vi "observacao_0MQ.vi"() -> ()   [LabVIEW 2012, in "Shared_160.lvlib"] (continued)
                    n1919 = property on="Sent_EspLampCass" class="Bool (strict)"("Disabled"=w2415) -> ()  [unwired: 2 in, 2 out]
                    n1920 = property on="Ne" class="Bool (strict)"("Disabled"=w2415) -> ()  [unwired: 2 in, 2 out]
                    n1921 = property on="He-Ar" class="Bool (strict)"("Disabled"=w2415) -> ()  [unwired: 2 in, 2 out]
                    n1922 = Add(x=w2416, y=u8 4) -> (x+y=w2418:u8)
                    n1923 = Greater Or Equal?(x=w2418, y=u8 100 ("x")) -> (x >= y?=w2419:bool)
                    n1924 = case shown="True" w2419 {
                      selector: w2419 -> [_ w2423]
                      tunnel: w2418 -> [w2422 _]
                      frame False {
                        n1925 = local write "SlideEcass"(w2422) -> ()
                        n1926 = property on="SlideEcass" class="Slide (strict)"("Fill Color"=u32 16750950 ("color(black)")) -> ()  [unwired: 2 in, 2 out]
                      }
                      frame True {
                        n1927 = local write "SlideEcass"(u8 92 ("Slide")) -> ()
                        n1928 = property on="stopEcass" class="Bool"("Visible"=w2423) -> ()  [unwired: 2 in, 2 out]
                        n1929 = property on="SlideEcass" class="Slide (strict)"("Fill Color"=u32 16724787 ("color(black)")) -> ()  [unwired: 2 in, 2 out]
                      }
                    }
                  }
                }
              }
              frame "Eucalyp." {
                # "Eucalyptus"
              }
              frame "Cam 1" {
                w2467 = 10
                w2474 = u16 15 items=["Alarme", "Atencao", "Erro", "Ocupado", "PosSecund", "PosConj#3", "MovFoco", "MovCjto#3", "Mov#4", "Mov#3", "Mov#2", "EspLamp", "HE", "NE", "EspLampRepouso", "EspLampCalibra"] ("NomeStatus")
                w2475 = u16 14 items=["Alarme", "Atencao", "Erro", "Ocupado", "PosSecund", "PosConj#3", "MovFoco", "MovCjto#3", "Mov#4", "Mov#3", "Mov#2", "EspLamp", "HE", "NE", "EspLampRepouso", "EspLampCalibra"] ("NomeStatus")
                w2476 = u16 11 items=["Alarme", "Atencao", "Erro", "Ocupado", "PosSecund", "PosConj#3", "MovFoco", "MovCjto#3", "Mov#4", "Mov#3", "Mov#2", "EspLamp", "HE", "NE", "EspLampRepouso", "EspLampCalibra"] ("NomeStatus")
                # "MUDANÇA:\nDESABILITA COMANDOS\nDE MOV. DO ESPELHO.\nRemover na implantação\ndefinitiva da CAM1."
                # "CAM 1"
                n1930 = event shown="[1] \"Mover/Parar\": Value Change" {
                  selector: _ -> [_ _ _ _]
                  dyn-events: _ -> [_ _ _ _]
                  timeout: w2467 -> [_ _ _ _]
                  tunnel: ["timeout" ("Comando") w2493 w2499 w2505] -> w2460
                  event Timeout {
                    n1931 = event-data() -> ()  [unwired: 1 in, 2 out]
                  }
                  event "Mover/Parar": Value Change {
                    w2495 = u16 3 items=["ZERO", "AH", "DEC", "TUBO", "CUP"] ("Controlador")
                    n1932 = event-data() -> ("NewVal"=w2496:bool)  [unwired: 1 in, 4 out]
                    n1933 = case shown="True" w2496 {
                      tunnel: ["PARAR" ("Comando") "GIRAR" ("Comando")] -> w2493
                      frame False {
                      }
                      frame True {
                      }
                    }
                    n1934 = call "Monta Comando.vi"("Comando"=w2493, "Dispositivo"="ESP_CAMP", "Controlador"=w2495) -> ()  [unwired: 4 in, 3 out]
                  }
                  event "Sentido": Value Change {
                    w2500 = u16 3 items=["ZERO", "AH", "DEC", "TUBO", "CUP"] ("Controlador")
                    n1935 = event-data() -> ("NewVal"=w2502:bool)  [unwired: 1 in, 4 out]
                    n1936 = case shown="False" w2502 {
                      tunnel: ["RECUAR" "AVANCAR"] -> w2499
                      frame False {
                      }
                      frame True {
                      }
                    }
                    n1937 = call "Monta Comando.vi"("Comando"=w2499, "Dispositivo"="ESP_CAMP", "Controlador"=w2500) -> ()  [unwired: 4 in, 3 out]
                  }
                  event "Velocidade": Value Change {
                    w2507 = u16 3 items=["ZERO", "AH", "DEC", "TUBO", "CUP"] ("Controlador")
                    n1938 = event-data() -> ("NewVal"=w2508:bool)  [unwired: 1 in, 4 out]
                    n1939 = case shown="True" w2508 {
                      tunnel: ["AUMENTAR" "DIMINUIR"] -> w2505
                      frame False {
                      }
                      frame True {
                      }
                    }
                    n1940 = call "Monta Comando.vi"("Comando"=w2505, "Dispositivo"="ESP_CAMP", "Controlador"=w2507) -> ()  [unwired: 4 in, 3 out]
                  }
                }
                "Comando" <- w2460
                n1941 = event shown="[1] \"Sent_EspDesvFeixe\": Value Change" {
                  selector: _ -> [_ _ _]
                  dyn-events: _ -> [_ _ _]
                  timeout: w2467 -> [_ _ _]
                  event Timeout {
                    n1942 = event-data() -> ()  [unwired: 1 in, 2 out]
                  }
                  event "Sent_EspDesvFeixe": Value Change {
                    n1943 = event-data() -> ()  [unwired: 1 in, 4 out]
                    n1944 = case shown="1" "Disabled" {
                      tunnel: ["RECUAR" ("Comando") "AVANCAR" ("Comando")] -> w2514
                      tunnel: ["ESP_LAMP" ("Dispositivo") "ESP_LAMP" ("Dispositivo")] -> w2513
                      frame 0, Default {
                        # "Case False (Default) em\noperação normal, com o\nbotão Sent_EspDesvFeixe\nligado ao ? deste case."
                      }
                      frame 1 {
                        # "CaseTrue. Cf. nota no case 0"
                        n1945 = property on="SlideCam1" class="Slide (strict)"("Visible"=TRUE) -> ()  [unwired: 2 in, 2 out]
                        n1946 = property on="stopCam1" class="Bool"("Visible"=FALSE) -> ()  [unwired: 2 in, 2 out]
                        "SlideCam1" <- u8 5 ("Slide 2")
                      }
                    }
                    n1947 = case shown="True" "Case Constant\n(See Context Help) 9" {
                      tunnel: w2514 -> [_ w2517]
                      tunnel: w2513 -> [_ w2516]
                      frame False {
                      }
                      frame True {
                        w2515 = u16 3 items=["ZERO", "AH", "DEC", "TUBO", "CUP"] ("Controlador")
                        n1948 = call "Monta Comando.vi"("Comando"=w2517, "Dispositivo"=w2516, "Controlador"=w2515) -> ()  [unwired: 4 in, 3 out]
                      }
                    }
                  }
                  event "Go_filtro": Value Change {
                    n1949 = event-data() -> ()  [unwired: 1 in, 6 out]
                    n1950 = case shown="True" "Go_filtro" {
                      frame False {
                      }
                      frame True {
                        (unwired) "ZERO: Porta serial da CAM1"
                        w2526 = u16 0 items=["ZERO", "AH", "DEC", "TUBO", "CUP"] ("Controlador")
                        n1951 = call "Monta Comando.vi"("Set Point"="Filtro", "Controlador"=w2526) -> ()  [unwired: 5 in, 3 out]
                      }
                    }
                  }
                }
                n1952 = case shown="False" "Sentido" {
                  tunnel: [TRUE FALSE] -> w2465
                  tunnel: [FALSE TRUE] -> w2464
                  frame False {
                  }
                  frame True {
                  }
                }
                "Recuar" <- w2465
                "Avancar" <- w2464
                n1953 = case shown="False" "Velocidade" {
                  tunnel: [TRUE FALSE] -> w2462
                  tunnel: [FALSE TRUE] -> w2461
                  frame False {
                  }
                  frame True {
                  }
                }
                "Rapido" <- w2462
                "Lento" <- w2461
                n1954 = call "Bit Status TUBO.vi"("NomeStatus"=w2476) -> ("StatBit"=w2473:bool)
                n1955 = call "Bit Status TUBO.vi"("NomeStatus"=w2475) -> ("StatBit"=w2472:bool)
                n1956 = call "Bit Status TUBO.vi"("NomeStatus"=w2474) -> ("StatBit"=w2471:bool)
                n1957 = Not(x=w2473) -> (.not. x?=w2482:bool)
                n1958 = And(x=w2473, y=w2472) -> (x .and. y?=w2478:bool)
                "LedRepCam1" <- w2478
                n1959 = Or(x=w2472, y=w2471) -> (x .or. y?=w2483:bool)
                n1960 = And(x=w2473, y=w2471) -> (x .and. y?=w2477:bool)
                "LedCalCam1" <- w2477
                n1961 = property on="SlideCam1" class="Slide (strict)"() -> ("Visible"=w2480:bool)  [unwired: 2 in, 2 out]
                n1962 = Or(x=w2478, y=w2477) -> (x .or. y?=w2481:bool)
                n1963 = And(x=w2482, y=w2483) -> (x .and. y?=w2469:bool)
                n1964 = And(x="Case Constant\n(See Context Help) 10", y=w2469) -> (x .and. y?=w2470:bool)
                n1965 = case shown="True" "Case Constant\n(See Context Help) 10" {
                  frame False {
                  }
                  frame True {
                    w2541 = FALSE
                    w2544 = u16 3 items=["ZERO", "AH", "DEC", "TUBO", "CUP"] ("Controlador")
                    w2542 = u8 0 ("Disabled")
                    n1966 = call "Monta Comando.vi"("Comando"="DESLIGAR", "Dispositivo"="ESP_LAMP", "Controlador"=w2544) -> ()  [unwired: 4 in, 3 out]
                    n1967 = property on="Sent_EspDesvFeixe" class="Bool (strict)"("Disabled"=w2542) -> ()  [unwired: 2 in, 2 out]
                    n1968 = property on="Go_filtro" class="Bool"("Disabled"=w2542) -> ()  [unwired: 2 in, 2 out]
                    n1969 = property on="stopCam1" class="Bool"("Visible"=w2541) -> ()  [unwired: 2 in, 2 out]
                    n1970 = property on="SlideCam1" class="Slide (strict)"("Visible"=w2541) -> ()  [unwired: 2 in, 2 out]
                  }
                }
                n1971 = case shown="True" w2470 {
                  frame False {
                  }
                  frame True {
                    w2529 = u8 2 ("Disabled")
                    n1972 = local read "SlideCam1"() -> (w2528:u8)
                    n1973 = Add(x=w2528, y=u8 5) -> (x+y=w2530:u8)
                    n1974 = property on="Sent_EspDesvFeixe" class="Bool (strict)"("Disabled"=w2529) -> ()  [unwired: 2 in, 2 out]
                    n1975 = property on="Go_filtro" class="Bool"("Disabled"=w2529) -> ()  [unwired: 2 in, 2 out]
                    n1976 = Greater Or Equal?(x=w2530, y=u8 100 ("x")) -> (x >= y?=w2532:bool)
                    n1977 = case shown="True" w2532 {
                      selector: w2532 -> [_ w2536]
                      tunnel: w2530 -> [w2534 _]
                      frame False {
                        n1978 = local write "SlideCam1"(w2534) -> ()
                        n1979 = property on="SlideCam1" class="Slide (strict)"("Fill Color"=u32 16750950 ("color(black)")) -> ()  [unwired: 2 in, 2 out]
                      }
                      frame True {
                        n1980 = property on="stopCam1" class="Bool"("Visible"=w2536) -> ()  [unwired: 2 in, 2 out]
                        n1981 = local write "SlideCam1"(u8 90 ("Slide 2")) -> ()
                        n1982 = property on="SlideCam1" class="Slide (strict)"("Fill Color"=u32 16724787 ("color(black)")) -> ()  [unwired: 2 in, 2 out]
                      }
                    }
                  }
                }
                n1983 = And(x=w2480, y=w2481) -> (x .and. y?=w2479:bool)
                n1984 = case shown="True" w2479 {
                  frame False {
                  }
                  frame True {
                    w2540 = u8 0 ("Disabled")
                    n1985 = property on="Go_filtro" class="Bool"("Disabled"=w2540) -> ()  [unwired: 2 in, 2 out]
                    n1986 = property on="Sent_EspDesvFeixe" class="Bool (strict)"("Disabled"=w2540) -> ()  [unwired: 2 in, 2 out]
                    n1987 = property on="SlideCam1" class="Slide (strict)"("Visible"=FALSE) -> ()  [unwired: 2 in, 2 out]
                  }
                }
              }
              frame "Cam 2" {
                # "Cam 2"
              }
              frame "Cam IV." {
                # "Cam IV"
              }
              frame "Polarim." {
                # "Polarimetro"
              }
              frame "Fotrap" {
                # "Fotrap"
              }
              frame "Coude", Default {
                # "COUDE"
                n1988 = stacked-sequence {
                  frame #0 {
                    w2548 = u16 5 items=["Alarme", "Atencao", "Erro", "Ocupado", "Stop#3", "Cass#3", "MovFoco", "PosSecund", "Mov#2", "Mov#3", "Mov#4", "EspLamp", "HE", "NE", "EspLampRepouso", "EspLampCalibra"] ("NomeStatus")
                    w2547 = u16 7 items=["Alarme", "Atencao", "Erro", "Ocupado", "Stop#3", "Cass#3", "MovFoco", "PosSecund", "Mov#2", "Mov#3", "Mov#4", "EspLamp", "HE", "NE", "EspLampRepouso", "EspLampCalibra"] ("NomeStatus")
                    n1989 = local read "EspAtual"() -> (w2550:string)
                    n1990 = case shown="\"A\"" w2550 {
                      frame "X", Default {
                        w2551 = FALSE
                        n1991 = local write "ledVisivel"(w2551) -> ()
                        n1992 = local write "ledAzul"(w2551) -> ()
                        n1993 = local write "ledVermelho"(w2551) -> ()
                      }
                      frame "M" {
                        w2552 = FALSE
                        n1994 = local write "ledAzul"(w2552) -> ()
                        n1995 = local write "ledVermelho"(w2552) -> ()
                        n1996 = local write "ledVisivel"(w2552) -> ()
                      }
                      frame "A" {
                        # "Espelho A --> Azul\nEspelho B --> Visível\nEspelho C --> Vermelho"
                        n1997 = local write "ledVermelho"(FALSE) -> ()
                        n1998 = local write "ledVisivel"(FALSE) -> ()
                        n1999 = local write "ledAzul"(TRUE) -> ()
                      }
                      frame "B" {
                        # "Espelho A --> Azul\nEspelho B --> Visível\nEspelho C --> Vermelho"
                        n2000 = local write "ledVermelho"(FALSE) -> ()
                        n2001 = local write "ledVisivel"(TRUE) -> ()
                        n2002 = local write "ledAzul"(FALSE) -> ()
                      }
                      frame "C" {
                        # "Espelho A --> Azul\nEspelho B --> Visível\nEspelho C --> Vermelho"
                        n2003 = local write "ledVermelho"(TRUE) -> ()
                        n2004 = local write "ledVisivel"(FALSE) -> ()
                        n2005 = local write "ledAzul"(FALSE) -> ()
                      }
                    }
                    n2006 = call "Bit Status TUBO.vi"("NomeStatus"=w2548) -> ("StatBit"=→"Cjto_3":bool)
                    n2007 = call "Bit Status TUBO.vi"("NomeStatus"=w2547) -> ("StatBit"=→"PosSecundario":bool)
                  }
                  frame #1 {
                    w2572 = u16 5 items=["Alarme", "Atencao", "Erro", "Ocupado", "Stop#3", "Cass#3", "MovFoco", "PosSecund", "Mov#2", "Mov#3", "Mov#4", "EspLamp", "HE", "NE", "EspLampRepouso", "EspLampCalibra"] ("NomeStatus")
                    w2577 = u16 8 items=["Alarme", "Atencao", "Erro", "Ocupado", "Stop#3", "Cass#3", "MovFoco", "PosSecund", "Mov#2", "Mov#3", "Mov#4", "EspLamp", "HE", "NE", "EspLampRepouso", "EspLampCalibra"] ("NomeStatus")
                    w2578 = u16 9 items=["Alarme", "Atencao", "Erro", "Ocupado", "Stop#3", "Cass#3", "MovFoco", "PosSecund", "Mov#2", "Mov#3", "Mov#4", "EspLamp", "HE", "NE", "EspLampRepouso", "EspLampCalibra"] ("NomeStatus")
                    w2579 = u16 10 items=["Alarme", "Atencao", "Erro", "Ocupado", "Stop#3", "Cass#3", "MovFoco", "PosSecund", "Mov#2", "Mov#3", "Mov#4", "EspLamp", "HE", "NE", "EspLampRepouso", "EspLampCalibra"] ("NomeStatus")
                    w2590 = u16 4 items=["Alarme", "Atencao", "Erro", "Ocupado", "Stop#3", "Cass#3", "MovFoco", "PosSecund", "Mov#2", "Mov#3", "Mov#4", "EspLamp", "HE", "NE", "EspLampRepouso", "EspLampCalibra"] ("NomeStatus")
                    w2591 = u16 3 items=["Alarme", "Atencao", "Erro", "Ocupado", "Stop#3", "Cass#3", "MovFoco", "PosSecund", "Mov#2", "Mov#3", "Mov#4", "EspLamp", "HE", "NE", "EspLampRepouso", "EspLampCalibra"] ("NomeStatus")
                    # "CJTO#3 EM \nMOVIMENTO"
                    n2008 = local read "PosSecundario"() -> (w2570:bool)
                    n2009 = call "Bit Status TUBO.vi"("NomeStatus"=w2572) -> ("StatBit"=w2569:bool)
                    n2010 = call "Bit Status TUBO.vi"("NomeStatus"=w2590) -> ("StatBit"=w2568:bool)
                    n2011 = call "Bit Status TUBO.vi"("NomeStatus"=w2591) -> ("StatBit"=w2566:bool)
                    n2012 = call "Bit Status TUBO.vi"("NomeStatus"=w2577) -> ("StatBit"=w2583:bool)
                    "#2" <- w2583
                    n2013 = call "Bit Status TUBO.vi"("NomeStatus"=w2578) -> ("StatBit"=w2582:bool)
                    "#3" <- w2582
                    n2014 = call "Bit Status TUBO.vi"("NomeStatus"=w2579) -> ("StatBit"=w2581:bool)
                    "#4" <- w2581
                    n2015 = Not Equal?(x=w2570, y=w2569) -> (x != y?=w2571:bool)
                    n2016 = Not(x=w2568) -> (.not. x?=w2564:bool)
                    n2017 = And(x=w2571, y=w2568) -> (x .and. y?=w2565:bool)
                    n2018 = Compound Arithmetic op=OR(w2583, w2582, w2581) -> (w2580:bool)
                    n2019 = Compound Arithmetic op=OR(w2565, w2564, w2566) -> (w2567:bool)
                    n2020 = property on="Cjto_3" class="Bool (strict)"("Blinking"=w2565) -> ()  [unwired: 2 in, 2 out]
                    n2021 = property on="PosSecundario" class="Bool (strict)"("Blinking"=w2565) -> ()  [unwired: 2 in, 2 out]
                    n2022 = case shown="True" w2567 {
                      tunnel: [T6."Page Enabled" ("Page Enabled State") T6."Page Disabled" ("Page Enabled State")] -> w2562
                      tunnel: [u8 0 ("Disabled") u8 2 ("Disabled")] -> w2576
                      frame False {
                      }
                      frame True {
                      }
                    }
                    n2023 = property on="MENSAGEM" class="Str"("Visible"=w2564, "Blinking"=w2564) -> ()  [unwired: 2 in, 2 out]
                    n2024 = case shown="True" w2580 {
                      tunnel: w2576 -> [w2595 _]
                      tunnel: [w2595 u8 2 ("Disabled")] -> w2575
                      tunnel: [FALSE TRUE] -> w2574
                      tunnel: [FALSE ("Blinking") TRUE ("Blinking")] -> w2573
                      frame False {
                        n2025 = local write "MENSAGEM 2"("EM MOVIMENTO" ("MENSAGEM 2")) -> ()
                      }
                      frame True {
                        n2026 = local read "EndTime"() -> (w2604:u32)
                        n2027 = Tick Count (ms)() -> (millisecond timer value=w2603:u32)
                        n2028 = Subtract(x=w2604, y=w2603) -> (x-y=w2602:u32)
                        n2029 = Divide(x=w2602, y=u32 1000) -> (x/y=w2599:dbl)
                        n2030 = To Unsigned Long Integer(number=w2599) -> (unsigned 32bit integer=w2600:u32)
                        n2031 = Number To Decimal String(number=w2600) -> (decimal integer string=w2597:string)  [unwired: 1 in]
                        n2032 = Concatenate Strings("EM MOVIMENTO " ("MENSAGEM 2"), w2597) -> (w2598:string)
                        n2033 = local write "MENSAGEM 2"(w2598) -> ()
                      }
                    }
                    n2034 = property on="Setup, Pointing & Guiding" class="TabCtl (strict)"() -> ("Pages"=w2563:refnum<vi>[])  [unwired: 2 in, 2 out]
                    n2035 = Index Array(array=w2563, index=4) -> (element=w2586:refnum<vi>)
                    n2036 = Index Array(array=w2563, index=5) -> (element=w2589:refnum<vi>)
                    n2037 = property class="Page"(reference=w2586, "Page Enabled State"=w2562) -> ()  [unwired: 1 in, 2 out]
                    n2038 = property class="Page"(reference=w2589, "Page Enabled State"=w2562) -> ()  [unwired: 1 in, 2 out]
                    n2039 = case shown="False" w2570 {
                      tunnel: [u8 0 ("Disabled") w2610] -> w2585
                      tunnel: w2575 -> [w2608 _]
                      tunnel: [w2608 w2610] -> w2584
                      frame False {
                        # "COUDE"
                      }
                      frame True {
                        w2610 = u8 2 ("Disabled")
                        # "CASS"
                      }
                    }
                    n2040 = property on="MENSAGEM 2" class="Str"("Visible"=w2574, "Blinking"=w2573) -> ()  [unwired: 2 in, 2 out]
                    n2041 = property on="ledAzul" class="Bool (strict)"("Disabled"=w2585) -> ()  [unwired: 2 in, 2 out]
                    n2042 = property on="ledVisivel" class="Bool (strict)"("Disabled"=w2585) -> ()  [unwired: 2 in, 2 out]
                    n2043 = property on="ledVermelho" class="Bool (strict)"("Disabled"=w2585) -> ()  [unwired: 2 in, 2 out]
                    n2044 = property on="Radio Buttons" class="RadioBtnsControl (strict)"("Disabled"=w2585) -> ()  [unwired: 2 in, 2 out]
                    n2045 = property on="#2" class="Bool (strict)"("Disabled"=w2585) -> ()  [unwired: 2 in, 2 out]
                    n2046 = property on="#3" class="Bool (strict)"("Disabled"=w2585) -> ()  [unwired: 2 in, 2 out]
                    n2047 = property on="#4" class="Bool (strict)"("Disabled"=w2585) -> ()  [unwired: 2 in, 2 out]
                    n2048 = property on="Go_Coudé" class="Bool"("Disabled"=w2584) -> ()  [unwired: 2 in, 2 out]
                  }
                  frame #2 {
                    n2049 = case shown="True" "Go_Coudé" {
                      frame False {
                        w2616 = u16 2 items=["Alarme", "Atencao", "Erro", "Ocupado", "Stop#3", "Cass#3", "MovFoco", "PosSecund", "Mov#2", "Mov#3", "Mov#4", "EspLamp", "HE", "NE", "EspLampRepouso", "EspLampCalibra"] ("NomeStatus")
                        w2617 = u16 3 items=["Alarme", "Atencao", "Erro", "Ocupado", "Stop#3", "Cass#3", "MovFoco", "PosSecund", "Mov#2", "Mov#3", "Mov#4", "EspLamp", "HE", "NE", "EspLampRepouso", "EspLampCalibra"] ("NomeStatus")
                        # "TRATA ERROS DO CONTROLADOR"
                        n2050 = call "Bit Status TUBO.vi"("NomeStatus"=w2616) -> ("StatBit"=w2619:bool)
                        n2051 = call "Bit Status TUBO.vi"("NomeStatus"=w2617) -> ("StatBit"=w2621:bool)
                        n2052 = Not(x=w2621) -> (.not. x?=w2620:bool)
                        n2053 = And(x=w2619, y=w2620) -> (x .and. y?=w2618:bool)
                        n2054 = case shown="True" w2618 {
                          frame False {
                          }
                          frame True {
                            w2624 = u16 3 items=["ZERO", "AH", "DEC", "TUBO", "CUP"] ("Controlador")
                            n2055 = call "Monta Comando.vi"("Comando"="ERROS", "Dispositivo"="PROG" ("Comando"), "Controlador"=w2624) -> ()  [unwired: 4 in, 3 out]
                          }
                        }
                      }
                      frame True {
                        w2625 = u16 3 items=["ZERO", "AH", "DEC", "TUBO", "CUP"] ("Controlador")
                        # "Enviar comando de \nmudar Espelho ABC"
                        n2056 = local read "EspAtual"() -> (w2631:string)
                        n2057 = case shown="\"Visível\"" "Radio Buttons" {
                          tunnel: ["C" ("Comando") "A" ("Comando") "B" ("Comando")] -> w2626
                          tunnel: w2631 -> [w2634 w2640 w2645]
                          tunnel: [w2633 w2639 w2646] -> w2628
                          frame "Vermelho" {
                            n2058 = case shown="\"A\"" w2634 {
                              tunnel: [u32 0 u32 60000 u32 35000] -> w2633
                              frame "C", Default {
                              }
                              frame "B" {
                              }
                              frame "A" {
                              }
                            }
                          }
                          frame "Azul", Default {
                            n2059 = case shown="\"C\"" w2640 {
                              tunnel: [u32 0 u32 35000 u32 60000] -> w2639
                              frame "A", Default {
                              }
                              frame "B" {
                              }
                              frame "C" {
                              }
                            }
                          }
                          frame "Visível" {
                            n2060 = case shown="\"C\"" w2645 {
                              tunnel: [u32 0 u32 60000 u32 35000] -> w2646
                              frame "B", Default {
                              }
                              frame "A" {
                              }
                              frame "C" {
                              }
                            }
                          }
                        }
                        n2061 = Tick Count (ms)() -> (millisecond timer value=w2630:u32)
                        n2062 = Add(x=w2630, y=w2628) -> (x+y=→"EndTime":u32)
                        n2063 = call "Monta Comando.vi"("Comando"=w2626, "Dispositivo"="ESPELHO" ("Comando"), "Controlador"=w2625) -> ()  [unwired: 4 in, 3 out]
                      }
                    }
                  }
                  frame #3 {
                    w2657 = 360.0
                    w2662 = 6.283185307179586
                    n2064 = global read "Global_Telescopio.vi" "guide_ang"() -> (w2672:string)
                    n2065 = global read "Global_Telescopio.vi" "guide_nor"() -> (w2673:string)
                    n2066 = global read "Global_Telescopio.vi" "AH_now"() -> (w2669:dbl)
                    n2067 = global read "Global_Telescopio.vi" "delta_now"() -> (w2670:dbl)
                    n2068 = Add(x=w2669, y=w2670) -> (x+y=w2661:dbl)
                    n2069 = Fract/Exp String To Number(string=w2672) -> (number=w2668:dbl)  [unwired: 3 in, 1 out]
                    n2070 = Fract/Exp String To Number(string=w2673) -> (number=w2671:dbl)  [unwired: 3 in, 1 out]
                    n2071 = Quotient & Remainder(x=w2661, y=w2662) -> (x-y*floor(x/y)=w2664:dbl)  [unwired: 1 out]
                    n2072 = Add(x=w2668, y=w2671) -> (x+y=w2653:dbl)
                    n2073 = Less Than 0?(x=w2664) -> (x < 0?=w2666:bool)
                    n2074 = case shown="True" w2666 {
                      tunnel: w2664 -> [w2674 w2677]
                      tunnel: [w2674 w2675] -> w2663
                      tunnel: w2662 -> [_ w2676]
                      frame False {
                      }
                      frame True {
                        n2075 = Add(x=w2677, y=w2676) -> (x+y=w2675:dbl)
                      }
                    }
                    n2076 = Add(x=124.0, y=w2653) -> (x+y=w2652:dbl)
                    n2077 = Multiply(x=w2663, y=57.29577951 ("x*y")) -> (x*y=w2660:dbl)
                    n2078 = Subtract(x=98.2, y=w2660) -> (x-y=w2659:dbl)
                    n2079 = Add(x=w2652, y=w2659) -> (x+y=w2656:dbl)
                    n2080 = Quotient & Remainder(x=w2656, y=w2657) -> (floor(x/y)=w2658:dbl)  [unwired: 1 out]
                    n2081 = Multiply(x=w2658, y=w2657) -> (x*y=w2655:dbl)
                    n2082 = Subtract(x=w2656, y=w2655) -> (x-y=→"Ang. Fenda":dbl)
                  }
                  frame #4 {
                    # "90"
                    # "270"
                    # "180"
                    # "0"
                    n2083 = event shown="[10] \"IronArc\": Value Change" {
                      selector: _ -> [_ _ _ _ _ _ _ _ _ _ _]
                      dyn-events: _ -> [_ _ _ _ _ _ _ _ _ _ _]
                      timeout: 10 -> [_ _ _ _ _ _ _ _ _ _ _]
                      event Timeout {
                        n2084 = event-data() -> ()  [unwired: 1 in, 2 out]
                        n2085 = stacked-sequence {
                          frame #0 {
                            n2086 = local read "parou 3"() -> (w2679:bool)
                            n2087 = case shown="True" w2679 {
                              frame False {
                              }
                              frame True {
                                n2088 = call "InstrumentControl.vi"("Input Message"="COUDE REDE POSICAO") -> ("Output Message"=w2682:string)  [unwired: 9 in, 1 out]
                                "Output Message" <- w2682
                                n2089 = Decimal String To Number(string=w2682) -> (number=w2681:i32)  [unwired: 2 in, 1 out]
                                n2090 = while {
                                shift-right: [w2685] -> w2680
                                shift-left: _ -> [w2689]
                                tunnel: w2681 -> [w2685]
                                stop <- TRUE stop-if-true
                                n2091 = Subtract(x=w2689, y=w2685) -> (x-y=w2688:i32)
                                n2092 = Absolute Value(x=w2688) -> (abs(x)=w2687:i32)
                                n2093 = Greater Or Equal?(x=w2687, y=1) -> (x >= y?=→"parou 3":bool)
                                }
                                "Posição Rede" <- w2680
                              }
                            }
                          }
                          frame #1 {
                            n2094 = local read "parou"() -> (w2692:bool)
                            n2095 = local read "parou 2"() -> (w2691:bool)
                            n2096 = case shown="True" w2691 {
                              frame False {
                              }
                              frame True {
                                # "Cada volta -> 10mm\nCada volta -> 4000counts\n1 count = 0,0025mm"
                                n2097 = call "InstrumentControl.vi"("Input Message"="COUDE ESPELHO POSICAO") -> ("Output Message"=w2699:string)  [unwired: 9 in, 1 out]
                                n2098 = Fract/Exp String To Number(string=w2699) -> (number=w2698:dbl)  [unwired: 3 in, 1 out]
                                n2099 = while {
                                shift-right: [w2711] -> w2694
                                shift-left: _ -> [w2712]
                                tunnel: w2698 -> [w2711]
                                tunnel: [w2707] -> w2693
                                stop <- TRUE stop-if-true
                                n2100 = Subtract(x=w2712, y=w2711) -> (x-y=w2710:dbl)
                                n2101 = Absolute Value(x=w2710) -> (abs(x)=w2709:dbl)
                                n2102 = Greater Or Equal?(x=w2709, y=0.02) -> (x >= y?=w2707:bool)
                                "parou 2" <- w2707
                                }
                                "Posição Espelho" <- w2694
                                n2103 = case shown="False" w2693 {
                                frame False {
                                n2104 = call "InstrumentControl.vi"("Input Message"="COUDE SERIAL CHAVEAR OFF") -> ()  [unwired: 9 in, 2 out]
                                }
                                frame True {
                                }
                                }
                                n2105 = Absolute Value(x=w2694) -> (abs(x)=w2695:dbl)
                                n2106 = Less Or Equal?(x=w2695, y=0.5) -> (x <= y?=w2697:bool)
                                n2107 = case shown="False" w2697 {
                                tunnel: w2695 -> [w2704 _]
                                frame False {
                                n2108 = Greater Or Equal?(x=w2704, y=34.5) -> (x >= y?=w2702:bool)
                                n2109 = case shown="True" w2702 {
                                frame False {
                                }
                                frame True {
                                n2110 = local write "Boolean"(TRUE ("Boolean")) -> ()
                                }
                                }
                                }
                                frame True {
                                n2111 = local write "Boolean"(FALSE ("Boolean")) -> ()
                                }
                                }
                              }
                            }
                            n2112 = case shown="True" w2692 {
                              frame False {
                              }
                              frame True {
                                n2113 = call "InstrumentControl.vi"("Input Message"="COUDE FENDA POSICAO") -> ("Output Message"=w2719:string)  [unwired: 9 in, 1 out]
                                n2114 = Fract/Exp String To Number(string=w2719) -> (number=w2718:dbl)  [unwired: 3 in, 1 out]
                                n2115 = Multiply(x=w2718, y=1000.0) -> (x*y=w2716:dbl)
                                n2116 = while {
                                shift-right: [w2726] -> w2715
                                shift-left: _ -> [w2727]
                                tunnel: w2716 -> [w2726]
                                tunnel: [w2722] -> w2714
                                stop <- TRUE stop-if-true
                                n2117 = Subtract(x=w2727, y=w2726) -> (x-y=w2725:dbl)
                                n2118 = Absolute Value(x=w2725) -> (abs(x)=w2724:dbl)
                                n2119 = Greater Or Equal?(x=w2724, y=1.0) -> (x >= y?=w2722:bool)
                                "parou" <- w2722
                                }
                                "Largura da Fenda 2" <- w2715
                                n2120 = case shown="False" w2714 {
                                frame False {
                                n2121 = call "InstrumentControl.vi"("Input Message"="COUDE SERIAL CHAVEAR OFF") -> ()  [unwired: 9 in, 2 out]
                                }
                                frame True {
                                }
                                }
                              }
                            }
                          }
                        }
                      }
                      event "Cathode": Value Change {
                        n2122 = event-data() -> ("NewVal"=w2729:bool)  [unwired: 1 in, 4 out]
                        n2123 = case shown="True" w2729 {
                          frame False {
                          }
                          frame True {
                            n2124 = flat-sequence {
                              frame #0 {
                                w2731 = FALSE ("NeAr")
                                n2125 = local write "Neon"(w2731) -> ()
                                n2126 = local write "Incand"(w2731) -> ()
                                n2127 = local write "Position"("Moving" ("Prisma Position")) -> ()
                                n2128 = call "Comando_Quick_Silver.vi"("COMANDO COMPLETO"="COUDE PRISMA MOVER 0" ("Input Message")) -> ()  [unwired: 2 in, 3 out]
                                n2129 = local write "IronArc"(w2731) -> ()
                              }
                              frame #1 {
                                n2130 = Wait (ms)(milliseconds to wait=u32 50) -> ()  [unwired: 1 out]
                              }
                              frame #2 {
                                n2131 = local write "Position"("Cathode" ("Prisma Position")) -> ()
                              }
                            }
                          }
                        }
                      }
                      event "Neon": Value Change {
                        n2132 = event-data() -> ("NewVal"=w2735:bool)  [unwired: 1 in, 4 out]
                        n2133 = case shown="True" w2735 {
                          frame False {
                          }
                          frame True {
                            n2134 = flat-sequence {
                              frame #0 {
                                w2737 = FALSE ("ThAr")
                                n2135 = local write "Cathode"(w2737) -> ()
                                n2136 = local write "Incand"(w2737) -> ()
                                n2137 = local write "Position"("Moving" ("Prisma Position")) -> ()
                                n2138 = call "Comando_Quick_Silver.vi"("COMANDO COMPLETO"="COUDE PRISMA MOVER 180" ("Input Message")) -> ()  [unwired: 2 in, 3 out]
                                n2139 = local write "IronArc"(w2737) -> ()
                              }
                              frame #1 {
                                n2140 = Wait (ms)(milliseconds to wait=u32 50) -> ()  [unwired: 1 out]
                              }
                              frame #2 {
                                n2141 = local write "Position"("Neon" ("Prisma Position")) -> ()
                              }
                            }
                          }
                        }
                      }
                      event "Incand": Value Change {
                        n2142 = event-data() -> ("NewVal"=w2741:bool)  [unwired: 1 in, 4 out]
                        n2143 = case shown="True" w2741 {
                          frame False {
                          }
                          frame True {
                            n2144 = flat-sequence {
                              frame #0 {
                                w2743 = FALSE ("ThAr")
                                n2145 = local write "Cathode"(w2743) -> ()
                                n2146 = local write "Neon"(w2743) -> ()
                                n2147 = local write "Position"("Moving" ("Prisma Position")) -> ()
                                n2148 = call "Comando_Quick_Silver.vi"("COMANDO COMPLETO"="COUDE PRISMA MOVER 270 " ("Input Message")) -> ()  [unwired: 2 in, 3 out]
                                n2149 = local write "IronArc"(w2743) -> ()
                              }
                              frame #1 {
                                n2150 = Wait (ms)(milliseconds to wait=u32 50) -> ()  [unwired: 1 out]
                              }
                              frame #2 {
                                n2151 = local write "Position"("Incand" ("Prisma Position")) -> ()
                              }
                            }
                          }
                        }
                      }
                      event Value Change {
                        n2152 = event-data() -> ("NewVal"=w2747:T4)  [unwired: 1 in, 4 out]
                        n2153 = case shown="True" w2747 {
                          frame False {
                          }
                          frame True {
                            n2154 = call "InstrumentControl.vi"("Input Message"="COUDE FENDA INICIAR") -> ()  [unwired: 9 in, 2 out]
                          }
                        }
                      }
                      event Value Change {
                        n2155 = event-data() -> ("NewVal"=w2749:T4)  [unwired: 1 in, 4 out]
                        n2156 = case shown="True" w2749 {
                          frame False {
                          }
                          frame True {
                            n2157 = call "Comando_Quick_Silver.vi"("COMANDO COMPLETO"="COUDE ESPELHO INICIAR" ("Input Message")) -> ()  [unwired: 2 in, 3 out]
                          }
                        }
                      }
                      event Value Change {
                        n2158 = event-data() -> ("NewVal"=w2751:T4)  [unwired: 1 in, 4 out]
                        n2159 = case shown="True" w2751 {
                          frame False {
                          }
                          frame True {
                            n2160 = call "InstrumentControl.vi"("Input Message"="COUDE PRISMA INICIAR") -> ()  [unwired: 9 in, 2 out]
                          }
                        }
                      }
                      event "Go Angulo de Difração": Value Change {
                        n2161 = event-data() -> ("NewVal"=w2753:bool)  [unwired: 1 in, 4 out]
                        n2162 = case shown="True" w2753 {
                          frame False {
                          }
                          frame True {
                            # "Envia comando para rede de difração"
                            n2163 = Number To Decimal String(number="Angulo da rede de difração") -> (decimal integer string=w2755:string)  [unwired: 1 in]
                            n2164 = Concatenate Strings("COUDE REDE MOVER ", w2755) -> (w2758:string)
                            n2165 = call "InstrumentControl.vi"("Input Message"=w2758) -> ()  [unwired: 9 in, 2 out]
                            n2166 = local write "parou 3"(TRUE ("parou 3")) -> ()
                          }
                        }
                      }
                      event "Go Largura da Fenda": Value Change {
                        n2167 = event-data() -> ("NewVal"=w2759:bool)  [unwired: 1 in, 4 out]
                        n2168 = case shown="True" w2759 {
                          frame False {
                          }
                          frame True {
                            n2169 = call "InstrumentControl.vi"("Input Message"="COUDE SERIAL CHAVEAR ON") -> ("error out"=w2761:errorcluster)  [unwired: 9 in, 1 out]
                            n2170 = Divide(x="Largura da Fenda", y=1000.0) -> (x/y=w2769:dbl)
                            n2171 = Number To Fractional String(use system decimal point (T)=FALSE, number=w2769, precision (6)=i16 6) -> (F-format string=w2763:string)  [unwired: 1 in]
                            n2172 = Concatenate Strings("COUDE FENDA MOVER ", w2763) -> (w2765:string)
                            n2173 = local write "parou"(TRUE ("parou")) -> ()
                            n2174 = call "InstrumentControl.vi"("error"=w2761, "Input Message"=w2765) -> ()  [unwired: 8 in, 2 out]
                          }
                        }
                      }
                      event "Prisma das Lâmpadas": Value Change {
                        n2175 = event-data() -> ("NewVal"=w2780:bool)  [unwired: 1 in, 4 out]
                        n2176 = case shown="False" w2780 {
                          tunnel: [0.0 ("y") 35.0 ("y")] -> w2778
                          frame False {
                            n2177 = local write "Boolean"(TRUE ("Boolean")) -> ()
                          }
                          frame True {
                            n2178 = local write "Boolean"(FALSE ("Boolean 2")) -> ()
                          }
                        }
                        n2179 = local write "parou 2"(TRUE ("parou 2")) -> ()
                        n2180 = call "InstrumentControl.vi"("Input Message"="COUDE SERIAL CHAVEAR ON") -> ("error out"=w2772:errorcluster)  [unwired: 9 in, 1 out]
                        n2181 = Number To Fractional String(use system decimal point (T)=FALSE, number=w2778, precision (6)=i16 6) -> (F-format string=w2773:string)  [unwired: 1 in]
                        n2182 = Concatenate Strings("COUDE ESPELHO MOVER ", w2773) -> (w2775:string)
                        n2183 = call "InstrumentControl.vi"("error"=w2772, "Input Message"=w2775) -> ()  [unwired: 8 in, 2 out]
                      }
                      event "IronArc": Value Change {
                        n2184 = event-data() -> ("NewVal"=w2785:bool)  [unwired: 1 in, 4 out]
                        n2185 = case shown="True" w2785 {
                          frame False {
                          }
                          frame True {
                            n2186 = flat-sequence {
                              frame #0 {
                                w2787 = FALSE ("ThAr")
                                n2187 = local write "Cathode"(w2787) -> ()
                                n2188 = local write "Neon"(w2787) -> ()
                                n2189 = call "Comando_Quick_Silver.vi"("COMANDO COMPLETO"="COUDE PRISMA MOVER 90 " ("Input Message")) -> ()  [unwired: 2 in, 3 out]
                                n2190 = local write "Position"("Moving" ("Prisma Position")) -> ()
                                n2191 = local write "Incand"(w2787) -> ()
                              }
                              frame #1 {
                                n2192 = Wait (ms)(milliseconds to wait=u32 50) -> ()  [unwired: 1 out]
                              }
                              frame #2 {
                                n2193 = local write "Position"("IronArc" ("Prisma Position")) -> ()
                              }
                            }
                          }
                        }
                      }
                    }
                  }
                }
              }
            }
          }
          frame "FOCUS" {
            w2827 = cluster{u32, u32}[] [] ("Colors [4]")
            w2828 = cluster{u32, u32}[] [] ("Colors [4]")
            # "ATUALIZA FOCO COM VALORES\nPUBLICADOS PELO FOCUSER160"
            # "dark(0)/bright(1)\n green"
            # "red(0)/greem(1)"
            # "ZeroMQ"
            # "T:  0x54      84\nC: 0x43       51\nS:  0x53      83\nP:  0x50      80\nD:  0x44      52\nClientId= 350"
            n2194 = global read "Global_Telescopio.vi" "queueSUB"() -> (w2822:refnum<queue>)
            n2195 = call "TX focus FOCO.vi"("Comando"="pos") -> ("pos (deg)"=→"old":dbl)  [unwired: 12 in, 2 out]
            n2196 = global read "Global_Telescopio.vi" "Focuser160"() -> (w2818:T11)
            n2197 = Get Queue Status(queue=w2822) -> (queue out=w2819:refnum<queue>, # elements in queue=w2821:i32)  [unwired: 2 in, 6 out]
            n2198 = Greater Than 0?(x=w2821) -> (x > 0?=w2820:bool)
            n2199 = case shown="True" w2820 {
              tunnel: w2819 -> [_ w2858]
              tunnel: w2818 -> [w2849 w2856]
              tunnel: [w2849 w2855] -> w2817
              frame False {
              }
              frame True {
                n2200 = Flush Queue(queue=w2858) -> (remaining elements=w2852:string[], error out=w2857:errorcluster)  [unwired: 1 in, 1 out]
                n2201 = Array Size(array=w2852) -> (size(s)=w2854:i32)
                "size(s)" <- w2854
                n2202 = Decrement(x=w2854) -> (x-1=w2853:i32)
                n2203 = Index Array(array=w2852, index=w2853) -> (element=w2851:string)
                "element" <- w2851
                n2204 = call "Focuser JSON to cluster.vi"("JSON status"=w2851) -> ("Focuser160"=w2850:T11)  [unwired: 10 in]
                n2205 = Select(t=w2856, s=w2857, f=w2850) -> (s? t:f=w2855:T11)
                n2206 = global write "Global_Telescopio.vi" "Focuser160"(w2855) -> ()
              }
            }
            n2207 = Unbundle By Name(w2817) -> ("alarm"=→"focuAlarm":bool, "cmd"=w2815:T12, "connected"=w2814:bool, "maxSpeed"=w2813:dbl, "position"=→"Foco":dbl, "error"=w2808:string, "homing"=→"focusHoming":bool, "initialized"=→"focusInitialized":bool, "isMoving"=→"focusMoving":bool)  [unwired: 1 out]
            "focusConnected" <- w2814
            n2208 = Unbundle By Name(w2815) -> ("clientId"=w2840:dbl)
            n2209 = Search and Replace String(replace all?=TRUE ("replace all? (F)"), input string=w2808, search string="\"") -> (result string=w2805:string)  [unwired: 5 in, 3 out]
            n2210 = Select(t=w2828, s=w2814, f=w2827) -> (s? t:f=w2825:cluster{u32, u32}[])
            n2211 = Select(t=w2828, s=w2814, f=w2827) -> (s? t:f=w2826:cluster{u32, u32}[])
            n2212 = property on="focusInitialized" class="Bool (strict)"("Colors [4]"=w2825) -> ()  [unwired: 2 in, 2 out]
            n2213 = property on="focuAlarm" class="Bool (strict)"("Colors [4]"=w2826) -> ()  [unwired: 2 in, 2 out]
            n2214 = case shown="True" "SetDefaultFocus" {
              frame False {
              }
              frame True {
                n2215 = global read "Global_Telescopio.vi" "Foco Instrumento"() -> (w2897:string)
                n2216 = Fract/Exp String To Number(string=w2897) -> (number=w2896:dbl)  [unwired: 3 in, 1 out]
                n2217 = local write "Setpoint"(w2896) -> ()
              }
            }
            n2218 = Empty String/Path?(string/path=w2805) -> (empty?=w2844:bool)
            n2219 = To Unsigned Word Integer(number=w2813) -> (unsigned 16bit integer=w2839:u16)
            n2220 = Not Equal?(x=350.0, y=w2840) -> (x != y?=w2799:bool)
            n2221 = Not Equal To 0?(x=w2840) -> (x != 0?=w2798:bool)
            n2222 = Not(x=w2814) -> (.not. x?=w2796:bool)
            n2223 = Number To Decimal String(number=w2839) -> (decimal integer string=w2837:string)  [unwired: 1 in]
            n2224 = And(x=w2799, y=w2798) -> (x .and. y?=w2800:bool)
            n2225 = Or(x=w2800, y=w2796) -> (x .or. y?=w2797:bool)
            n2226 = Multiply(x=w2813, y="Velocity") -> (x*y=w2793:dbl)
            n2227 = Concatenate Strings("(max = " ("string"), w2837, " u/s)" ("string")) -> (w2831:string)
            n2228 = Select(t="            Focus Status", s=w2844, f=w2805) -> (s? t:f=→"focusStatus":string)
            n2229 = Divide(x=w2793, y=100.0) -> (x/y=w2791:dbl)
            n2230 = Select(t=T5."Disabled and Grayed Out" ("Disabled"), s=w2797, f=T5."Enabled" ("Disabled")) -> (s? t:f=w2801:T5)
            n2231 = property on="Velocity" class="Slide (strict)"("Caption.Text"=w2831) -> ()  [unwired: 2 in, 2 out]
            n2232 = property on="focusGo" class="Bool"("Disabled"=w2801) -> ()  [unwired: 2 in, 2 out]
            n2233 = property on="focusHome" class="Bool"("DisabledEnum"=w2801) -> ()  [unwired: 2 in, 2 out]
            n2234 = property on="Focus -" class="Bool (strict)"("Disabled"=w2801) -> ()  [unwired: 2 in, 2 out]
            n2235 = property on="Focus +" class="Bool (strict)"("Disabled"=w2801) -> ()  [unwired: 2 in, 2 out]
            n2236 = Number To Decimal String(number=w2791) -> (decimal integer string=w2829:string)  [unwired: 1 in]
            n2237 = property on="Focus -" class="Bool (strict)"() -> ("BoolText.Text"=w2802:string)  [unwired: 2 in, 2 out]
            n2238 = property on="Focus +" class="Bool (strict)"() -> ("BoolText.Text"=w2803:string)  [unwired: 2 in, 2 out]
            n2239 = case shown="True" "focusHome" {
              frame False {
              }
              frame True {
                n2240 = global read "Global_Telescopio.vi" "transactionId0MQ"() -> (w2893:u64)
                n2241 = Increment(x=w2893) -> (x+1=w2894:u64)
                n2242 = global write "Global_Telescopio.vi" "transactionId0MQ"(w2894) -> ()
                n2243 = call "Focus PUSH.vi"("action"="HOME" ("controller"), "clientTransactionId"=w2893) -> ()  [unwired: 9 in, 1 out]
              }
            }
            n2244 = case shown="True" "focusStop" {
              frame False {
              }
              frame True {
                n2245 = global read "Global_Telescopio.vi" "transactionId0MQ"() -> (w2846:u64)
                n2246 = Increment(x=w2846) -> (x+1=w2847:u64)
                n2247 = call "Focus PUSH.vi"("action"="HALT" ("controller"), "clientTransactionId"=w2846) -> ()  [unwired: 9 in, 1 out]
                n2248 = global write "Global_Telescopio.vi" "transactionId0MQ"(w2847) -> ()
              }
            }
            n2249 = case shown="False" "Focus -" {
              tunnel: w2829 -> [w2860 w2868]
              tunnel: w2802 -> [w2859 w2867]
              frame True {
                n2250 = case shown="\"OFF\"" w2859 {
                  tunnel: w2860 -> [_ w2865]
                  frame "ON", Default {
                  }
                  frame "OFF" {
                    n2251 = global read "Global_Telescopio.vi" "transactionId0MQ"() -> (w2862:u64)
                    n2252 = Concatenate Strings("FOCUSIN=" ("controller"), w2865) -> (w2864:string)
                    n2253 = Increment(x=w2862) -> (x+1=w2863:u64)
                    n2254 = call "Focus PUSH.vi"("action"=w2864, "clientTransactionId"=w2862) -> ()  [unwired: 9 in, 1 out]
                    n2255 = global write "Global_Telescopio.vi" "transactionId0MQ"(w2863) -> ()
                    n2256 = property on="Focus -" class="Bool (strict)"("BoolText.Text"="ON") -> ()  [unwired: 2 in, 2 out]
                  }
                }
              }
              frame False {
                n2257 = case shown="\"ON\"" w2867 {
                  tunnel: w2868 -> [_ _]
                  frame "ON" {
                    n2258 = global read "Global_Telescopio.vi" "transactionId0MQ"() -> (w2870:u64)
                    n2259 = property on="Focus -" class="Bool (strict)"("BoolText.Text"="OFF") -> ()  [unwired: 2 in, 2 out]
                    n2260 = Increment(x=w2870) -> (x+1=w2871:u64)
                    n2261 = global write "Global_Telescopio.vi" "transactionId0MQ"(w2871) -> ()
                    n2262 = call "Focus PUSH.vi"("action"="HALT" ("controller"), "clientTransactionId"=w2870) -> ()  [unwired: 9 in, 1 out]
                  }
                  frame "OFF", Default {
                  }
                }
              }
            }
            n2263 = case shown="True" "focusGo" {
              frame False {
              }
              frame True {
                n2264 = global read "Global_Telescopio.vi" "transactionId0MQ"() -> (w2887:u64)
                n2265 = Number To Decimal String(number="Setpoint") -> (decimal integer string=w2891:string)  [unwired: 1 in]
                n2266 = Concatenate Strings("MOVE=" ("controller"), w2891) -> (w2889:string)
                n2267 = Increment(x=w2887) -> (x+1=w2888:u64)
                n2268 = global write "Global_Telescopio.vi" "transactionId0MQ"(w2888) -> ()
                n2269 = call "Focus PUSH.vi"("action"=w2889, "clientTransactionId"=w2887) -> ()  [unwired: 9 in, 1 out]
              }
            }
            n2270 = case shown="False" "Focus +" {
              tunnel: w2829 -> [w2874 w2882]
              tunnel: w2803 -> [w2873 w2881]
              frame True {
                n2271 = case shown="\"OFF\"" w2873 {
                  tunnel: w2874 -> [w2879 _]
                  frame "OFF" {
                    n2272 = global read "Global_Telescopio.vi" "transactionId0MQ"() -> (w2875:u64)
                    n2273 = property on="Focus +" class="Bool (strict)"("BoolText.Text"="ON") -> ()  [unwired: 2 in, 2 out]
                    n2274 = Concatenate Strings("FOCUSOUT=" ("controller"), w2879) -> (w2878:string)
                    n2275 = Increment(x=w2875) -> (x+1=w2876:u64)
                    n2276 = call "Focus PUSH.vi"("action"=w2878, "clientTransactionId"=w2875) -> ()  [unwired: 9 in, 1 out]
                    n2277 = global write "Global_Telescopio.vi" "transactionId0MQ"(w2876) -> ()
                  }
                  frame "ON", Default {
                  }
                }
              }
              frame False {
                n2278 = case shown="\"ON\"" w2881 {
                  tunnel: w2882 -> [_ _]
                  frame "ON" {
                    n2279 = global read "Global_Telescopio.vi" "transactionId0MQ"() -> (w2883:u64)
                    n2280 = property on="Focus +" class="Bool (strict)"("BoolText.Text"="OFF") -> ()  [unwired: 2 in, 2 out]
                    n2281 = Increment(x=w2883) -> (x+1=w2884:u64)
                    n2282 = global write "Global_Telescopio.vi" "transactionId0MQ"(w2884) -> ()
                    n2283 = call "Focus PUSH.vi"("action"="HALT" ("controller"), "clientTransactionId"=w2883) -> ()  [unwired: 9 in, 1 out]
                  }
                  frame "OFF", Default {
                  }
                }
              }
            }
          }
          frame "ROTATOR" {
            # "MUDANÇA 22/6/11:\nValor default passou a ser carregado no início deste VI."
            n2284 = case shown="True" "Set Rotator Angle" {
              frame False {
              }
              frame True {
                # "MUDANÇA 22/6/11:\nIncluída a formatação\nda string"
                n2285 = call "Formata_Numeros.vi"("Formato ex-> 7.2"="7.2", "Valor num"="New Angle") -> ("resulting string"=w2907:string)
                "Rotator Angle" <- w2907
                n2286 = global write "Global_Telescopio.vi" "guide_ang"(w2907) -> ()
              }
            }
            n2287 = global write "Global_Telescopio.vi" "Flag-Rotator"(FALSE ("Flag-Rotator")) -> ()
            n2288 = local read "Default Angle"() -> (w2900:string)
            n2289 = global read "Global_Telescopio.vi" "rotator_def"() -> (w2901:string)
            n2290 = Not Equal?(x=w2901, y=w2900) -> (x != y?=w2899:bool)
            n2291 = case shown="True" "SetRotatorDefAngle" {
              tunnel: w2900 -> [_ w2905]
              frame False {
              }
              frame True {
                n2292 = local write "Rotator Angle"(w2905) -> ()
                n2293 = global write "Global_Telescopio.vi" "guide_ang"(w2905) -> ()
              }
            }
            n2294 = case shown="True" w2899 {
              tunnel: w2901 -> [_ w2904]
              frame False {
              }
              frame True {
                n2295 = local write "Rotator Angle"(w2904) -> ()
                n2296 = global write "Global_Telescopio.vi" "guide_ang"(w2904) -> ()
                "Default Angle" <- w2904
              }
            }
          }
          frame "DOME" {
            w2922 = u16 6 items=["Alarme", "Atencao", "Erro", "Ocupado", "TBD", "LCB", "Trapeira", "Paravento", "DomoRap", "DomoCW", "DomoCCW", "TBD", "Em movimento", "TBD"] ("NomeStatus")
            w2926 = u16 3 items=["Alarme", "Atencao", "Erro", "Ocupado", "TBD", "LCB", "Trapeira", "Paravento", "DomoRap", "DomoCW", "DomoCCW", "TBD", "Em movimento", "TBD"] ("NomeStatus")
            # "MUDANÇA:\nO CW CCW comandos enviados ao controlador\nde girar e parar, estão escondidos. 26-01-2022"
            # "MUDANÇA:\nO RESET do uC CUP apaga o estado da trapeira (e paravento) o que compromote seu controle.\nNecessário implantar sensor de estado da trapeira."
            n2297 = disable-structure shown="Disabled" {
              frame Disabled {
                w2931 = TRUE  # CUP unlock enable
                # "Checa travamento CUP"
                n2298 = global read "Global_Telescopio.vi" "CupStartPos"() -> (w2933:i16)
                n2299 = global read "Global_Telescopio.vi" "RevCupTO"() -> (w2932:u32)
                n2300 = call "Checa destino cupula.vi"("Target"=w2933) -> ("moverCup"=w2936:bool)  [unwired: 6 in, 2 out]
                n2301 = call "TickTimeout.vi"("msInicial"=w2932, "msTimeout"=u32 8000) -> ("msTick"=w2938:u32, "Timeout"=w2934:bool)  [unwired: 1 out]
                n2302 = Compound Arithmetic op=AND(invert w2936, w2934, w2931) -> (w2937:bool)
                n2303 = case shown="True" w2936 {
                  tunnel: w2938 -> [_ w2944]
                  frame False {
                  }
                  frame True {
                    n2304 = global write "Global_Telescopio.vi" "RevCupTO"(w2944) -> ()
                    n2305 = local write "StatDome"("Moving" ("Status")) -> ()
